vi "PAQ_File_Read_TimeRange.vi"(8 "error in (no error)":errorcluster, 11 "FilePath":path) -> (0 "error out":errorcluster, 1 "TAGs":string[](array[string]), 2 "Tmin":timestamp, 3 "Tmax":timestamp)   [LabVIEW 2020]
doc: "Read min/max time of a PAQ file"
uses:
  DBAL-BIN.lvclass
panel:
  out "Fetched samples":i32
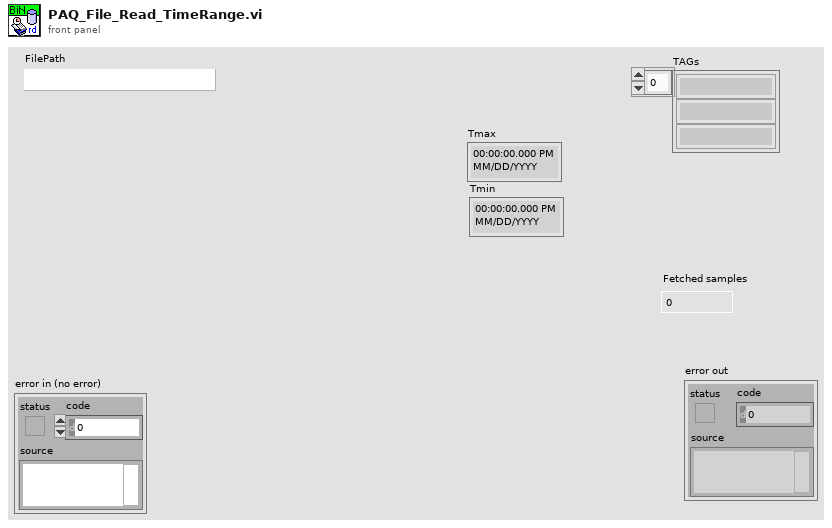
[diagram p1: front panel]
types:
  T1 = typedef "DBAL-BIN.lvclass/BINdata.ctl" = cluster{"time":dbl[], "TagsData":cluster{"data":dbl[], "max":dbl[], "min":dbl[], "status":u32[]}[]}
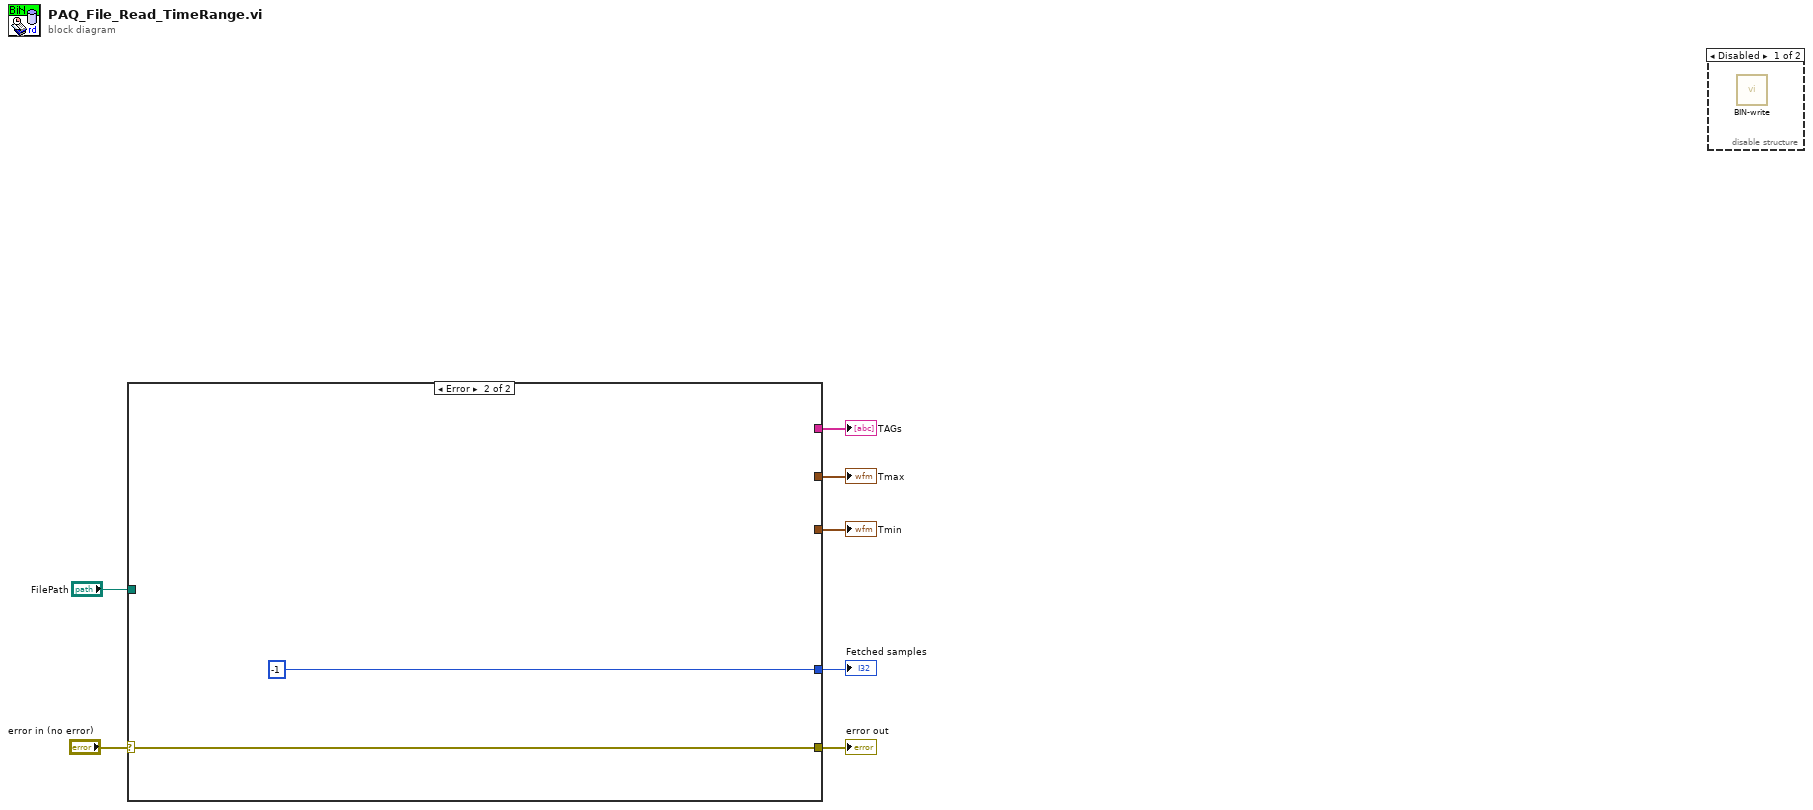
[diagram p0: block diagram]
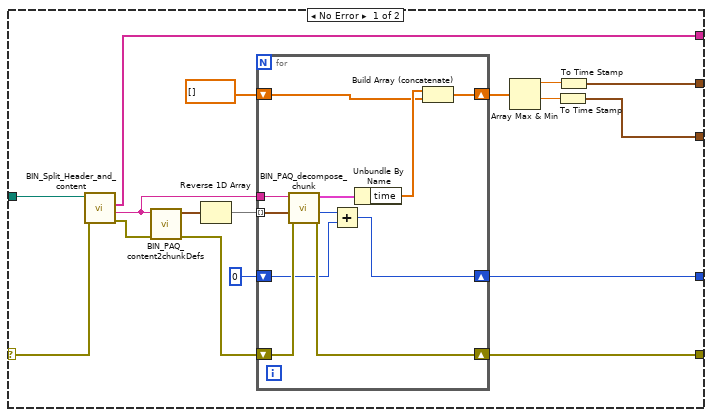
[diagram p3: hidden frame]
diagram:
  n1 = case shown="Error" "error in (no error)" {
    selector: "error in (no error)" -> [w24 w37]
    tunnel: [w20 w37] -> w6
    tunnel: "FilePath" -> [w14 _]
    tunnel: [w16 -1 ("Samples size")] -> w3
    tunnel: [w15 _] -> w4
    tunnel: [w9 _] -> w2
    tunnel: [w8 _] -> w1
    frame No Error {
      n2 = call "BIN_Split_Header_and_content.vi"("error in"=w24, "Path in"=w14) -> ("error out"=w23:errorcluster, "Content"=w22:string, "TAGs"=w15:string[])  [unwired: 5 in, 2 out]
      n3 = call "BIN_PAQ_content2chunkDefs.vi"("error in (no error)"=w23, "Content"=w22) -> ("error out"=w21:errorcluster, "Data segments"=w19:cluster{"Offset":u32, "Size":u32}[])  [unwired: 8 in]
      n4 = Reverse 1D Array(array=w19) -> (reversed array=w18:cluster{"Offset":u32, "Size":u32}[])
      n5 = for {
        tunnel: w18 -> [w35] mode=indexing
        tunnel: w22 -> [w34]
        shift-right: [w32] -> w20
        shift-left: w21 -> [w33]
        shift-right: [w27] -> w16
        shift-left: 0 ("Samples size") -> [w28]
        shift-right: [w25] -> w12
        shift-left: dbl[] [] ("time") -> [w26]
        n6 = call "BIN_PAQ_decompose_chunk.vi"("error in (no error)"=w33, "Offset"=w35, "Content"=w34) -> ("error out"=w32:errorcluster, "Samples size"=w29:i32, "PAQ_data"=w31:T1)  [unwired: 6 in]
        n7 = Add(x=w29, y=w28) -> (x+y=w27:i32)
        n8 = Unbundle By Name(w31) -> ("time"=w30:dbl[])
        n9 = Build Array (concatenate)(w30, w26) -> (w25:dbl[])
      }
      n10 = Array Max & Min(array=w12) -> (max value=w11:dbl, min value=w10:dbl)  [unwired: 2 out]
      n11 = To Time Stamp(1:w10) -> (0:w8:timestamp)
      n12 = To Time Stamp(1:w11) -> (0:w9:timestamp)
    }
    frame Error {
    }
  }
  "error out" <- w6
  "Fetched samples" <- w3
  "TAGs" <- w4
  "Tmax" <- w2
  "Tmin" <- w1
  n13 = disable-structure shown="Disabled" {
    frame Disabled {
      n14 = call "BIN-write.vi"() -> ()  [unwired: 11 in, 1 out]
    }
    frame Enabled {
    }
  }
